vi "conv.pretty.ob.cmd.to.cluster.vi"(11 "val.pretty.OrderBook.Commands.In":T3[](array[typedef]) {"side" items=["Buy"=102, "Sell"=131]; "orderId" format="%.0x"}) -> (3 "OrderBook.Commands.out":T1[](array[typedef]) {"symbol" format="%.0x"})   [LabVIEW 2020]
uses:
  fpga/common/orderbook.command.type.ctl
  fpga/common/orderbook.command.ctl
  types/val.pretty.orderbook.command.ctl
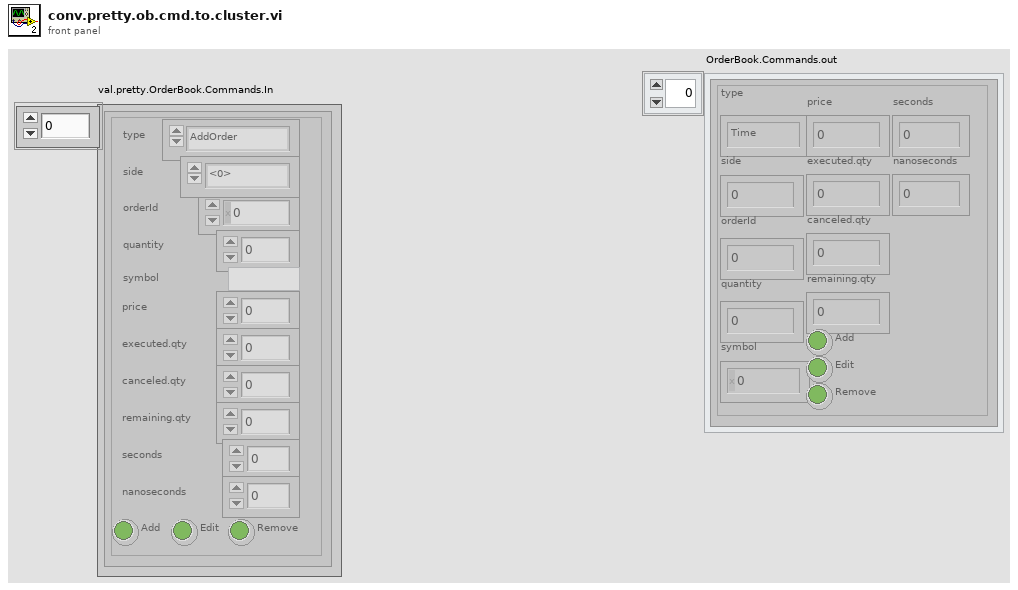
[diagram p1: front panel]
types:
  T1 = typedef "orderbook.command.ctl" = cluster{"type":T2, "side":u8, "orderId ":u64, "quantity":u32, "symbol":u64, "price":u64, "executed.qty":u32, "canceled.qty":u32, "remaining.qty":u32, "seconds":u64, "nanoseconds":u64, "Add":bool, "Edit":bool, "Remove":bool}
  T2 = typedef "orderbook.command.type.ctl" = enum8{"Time", "AddOrder", "OrderExecuted", "OrderExecutedAtPrice", "ReduceSize", "ModifyOrder", "DeleteOrder", "Get.Everything", "Get.All.Orders", "Get.Top"}
  T3 = typedef "val.pretty.orderbook.command.ctl" = cluster{"type":T2, "side":i16, "orderId ":u64, "quantity":u32, "symbol":string, "price":sgl, "executed.qty":u32, "canceled.qty":u32, "remaining.qty":u32, "seconds":u64, "nanoseconds":u64, "Add":bool, "Edit":bool, "Remove":bool}
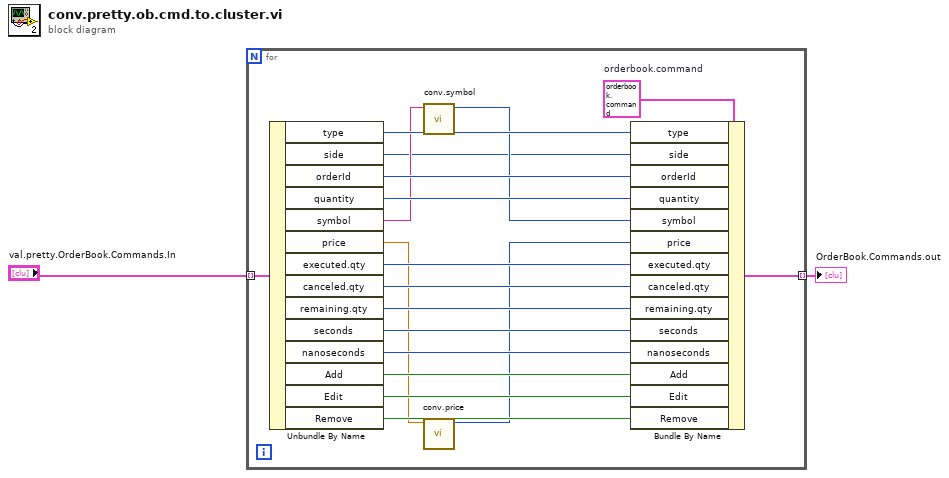
[diagram p0: block diagram]
diagram:
  n1 = for {
    tunnel: "val.pretty.OrderBook.Commands.In" -> [w20] mode=indexing
    tunnel: [w8] -> w1 mode=indexing
    w21 = T1 {"type"=enum."AddOrder", "side"=0, "orderId "=0, "quantity"=0, "symbol"=0, "price"=0, "executed.qty"=0, "canceled.qty"=0, "remaining.qty"=0, "seconds"=0, "nanoseconds"=0, "Add"=FALSE, "Edit"=FALSE, "Remove"=FALSE}  # orderbook.command
    n2 = Unbundle By Name(w20) -> ("type"=w19:T2, "side"=w5:i16, "orderId"=w18:u64, "quantity"=w9:u32, "symbol"=w7:string, "price"=w4:sgl, "executed.qty"=w10:u32, "canceled.qty"=w11:u32, "remaining.qty"=w12:u32, "seconds"=w13:u64, "nanoseconds"=w14:u64, "Add"=w15:bool, "Edit"=w16:bool, "Remove"=w17:bool)
    n3 = call "conv.symbol.vi"("symbol.in"=w7) -> ("symbol.out"=w6:u64)  [unwired: 10 in]
    n4 = call "conv.price.vi"("price.in"=w4) -> ("price.out"=w3:u64)  [unwired: 10 in]
    n5 = Bundle By Name(cluster=w21, "type"=w19, "side"=w5, "orderId"=w18, "quantity"=w9, "symbol"=w6, "price"=w3, "executed.qty"=w10, "canceled.qty"=w11, "remaining.qty"=w12, "seconds"=w13, "nanoseconds"=w14, "Add"=w15, "Edit"=w16, "Remove"=w17) -> (w8:T1)
  }
  "OrderBook.Commands.out" <- w1
